vi "VD-emptyBuffer.vi"(8 "error in (no error)":errorcluster, 11 "VD-LV-LiteVNA in":refnum<class "VD-LV-LiteVNA.lvclass">) -> (0 "error out":errorcluster, 1 "size(s)":i32, 2 "read buffer":T1 format="%x", 3 "VD-LV-LiteVNA out":refnum<class "VD-LV-LiteVNA.lvclass">, 4 "Remaining Bytes at Port":u32)   [LabVIEW 2020, in "VD-LV-LiteVNA.lvclass"]
uses:
  VD-LV-LiteVNA.lvclass
  hardware-protocol/serial/HP-S-data.ctl
  VD-LV-LiteVNA.lvclass/VD-LV-LiteVNA.ctl
  hardware-protocol/serial/HP-S-Serial.lvclass
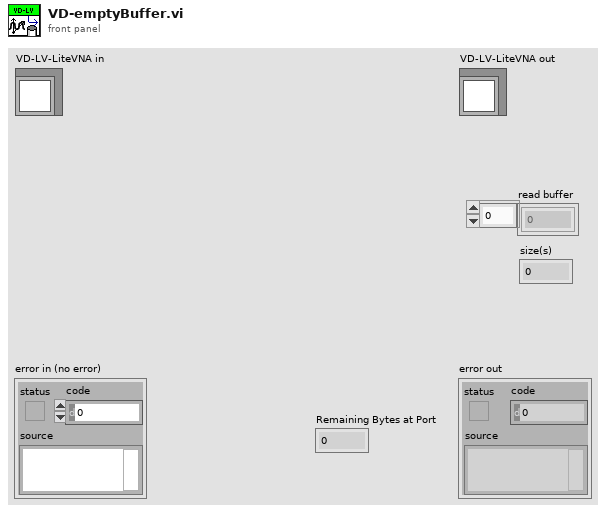
[diagram p1: front panel]
types:
  T1 = typedef "HP-S-Serial.lvclass/HP-S-data.ctl" = u8[]
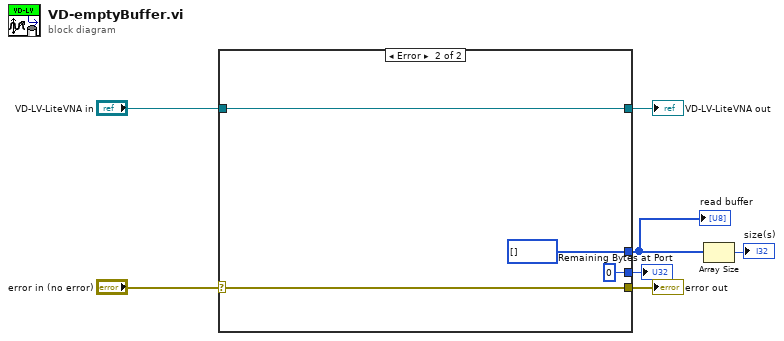
[diagram p0: block diagram]
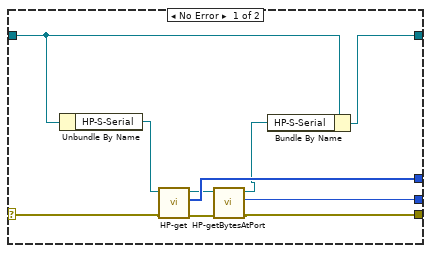
[diagram p2: hidden frame]
diagram:
  n1 = case shown="Error" "error in (no error)" {
    selector: "error in (no error)" -> [w14 w21]
    tunnel: [w8 w21] -> w6
    tunnel: [w16 w20] -> w4
    tunnel: "VD-LV-LiteVNA in" -> [w17 w20]
    tunnel: [w13 T1 [] ("read buffer")] -> w2
    tunnel: [w9 u32 0 ("Serial Settings:Number of Bytes at Serial Port")] -> w1
    frame No Error {
      n2 = Unbundle By Name(w17) -> ("HP-S-Serial"=w15:refnum<class "HP-S-Serial.lvclass">)
      n3 = call-dynamic "HP-get.vi"("error in (no error)"=w14, "HP-S-Serial in"=w15) -> ("error out"=w12:errorcluster, "read buffer"=w13:T1, "HP-S-Serial out"=w11:refnum<class "HP-S-Serial.lvclass">)  [unwired: 7 in]
      n4 = call-dynamic "HP-getBytesAtPort.vi"("error in (no error)"=w12, "HP-S-Serial in"=w11) -> ("error out"=w8:errorcluster, "Serial Settings:Number of Bytes at Serial Port"=w9:u32, "HP-S-Serial out"=w10:refnum<class "HP-S-Serial.lvclass">)  [unwired: 7 in]
      n5 = Bundle By Name(cluster=w17, "HP-S-Serial"=w10) -> (w16:refnum<class "VD-LV-LiteVNA.lvclass">)
    }
    frame Error {
    }
  }
  "error out" <- w6
  "VD-LV-LiteVNA out" <- w4
  "read buffer" <- w2
  "Remaining Bytes at Port" <- w1
  n6 = Array Size(array=w2) -> (size(s)=→"size(s)":i32)
